vi "Ramp to Zero.vi"(6 "Axis":T1, 8 "error in (no error)":errorcluster, 11 "Instrument.VRM in":refnum<class "Instrument.OxfordVRM.lvclass">) -> (0 "error out":errorcluster, 2 "Response":string, 3 "Instrument.VRM out":refnum<class "Instrument.OxfordVRM.lvclass">)   [LabVIEW 2019, in "Instrument.OxfordVRM.lvclass"]
uses:
  Instrument.OxfordVRM.lvclass
  C:/Program Files (x86)/National Instruments/LabVIEW 2019/user.lib/LevyLab/Levylab Instruments/SMOs/Instrument/Instrument.lvclass
  Typedefs/VRM Magnet Axis--Enum.ctl
  <instrlib>/Mercury iXX/Public/Libraries/Magnet/Controls/PSU Actions.ctl
  Typedefs/Instrument.VRM.Commands-enum.ctl
  Typedefs/VRM Action-Axis--Cluster.ctl
  <userlib>/LevyLab/Instrument Framework/SMOs/Instrument/Instrument.lvclass/Instrument.ctl
  c467e4a8-4b58-44aa-8f24-0652f0f40db9.vi
  c467e4a8-4b58-44aa-8f24-0652f0f40db9.vi/cb162148-aced-4026-a92a-8c3683a6e699.vi
  c467e4a8-4b58-44aa-8f24-0652f0f40db9.vi/cb162148-aced-4026-a92a-8c3683a6e699.vi/90903bc8-b2cf-450b-a3a9-0f5a5b9220d8.vi
  <userlib>/LevyLab/Instrument Framework/SMOs/Instrument/API/Send and Receive.vi
  c467e4a8-4b58-44aa-8f24-0652f0f40db9.vi/cb162148-aced-4026-a92a-8c3683a6e699.vi/90903bc8-b2cf-450b-a3a9-0f5a5b9220d8.vi/98039df1-7789-4232-8489-3644d3569676.vi
  c467e4a8-4b58-44aa-8f24-0652f0f40db9.vi/cb162148-aced-4026-a92a-8c3683a6e699.vi/90903bc8-b2cf-450b-a3a9-0f5a5b9220d8.vi/acf00810-0388-4f91-a2e6-f9b1b5e55ebd.vi
  <userlib>/LevyLab/Instrument Framework/SMOs/Instrument/API/Enum to String.vi
  <userlib>/LevyLab/Instrument Framework/SMOs/RemoteControl/API/Send and Receive.vi
  <vilib>/Utility/Data Type/Get Type Information.vi
  <vilib>/JDP Science/JSONtext/JSON text to Variant.vi
  <vilib>/JDP Science/JSONtext/LVClass Serializer/JSONtext LVClass Serializer.lvclass
  <instrlib>/Mercury iXX/Public/Libraries/Magnet.lvlib
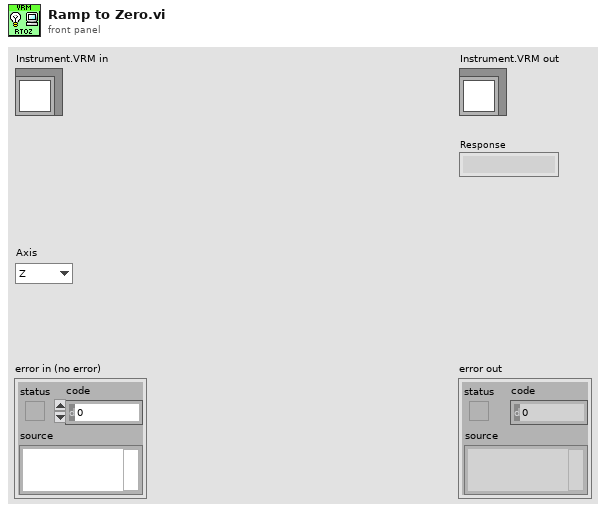
[diagram p1: front panel]
types:
  T1 = typedef "Instrument.OxfordVRM.lvclass/VRM Magnet Axis--Enum.ctl" = enum16{"Z", "X", "Y", "ALL"}
  T2 = typedef "Instrument.OxfordVRM.lvclass/VRM Action-Axis--Cluster.ctl" = cluster{"PSU Act Stat":T3, "Axis":T1}
  T3 = typedef "Mercury iXX.lvlib/Magnet.lvlib/PSU Actions.ctl" = string
  T4 = typedef "Instrument.OxfordVRM.lvclass/Instrument.VRM.Commands-enum.ctl" = enum16{"setAction", "setTarget", "setMagnetField", "getStatus", "getTarget", "getMagnetField"}
  T5 = cluster{"Holding":bool, "Ramp to Setpoint":bool, "Ramp to Zero":bool, "Clamp":bool}
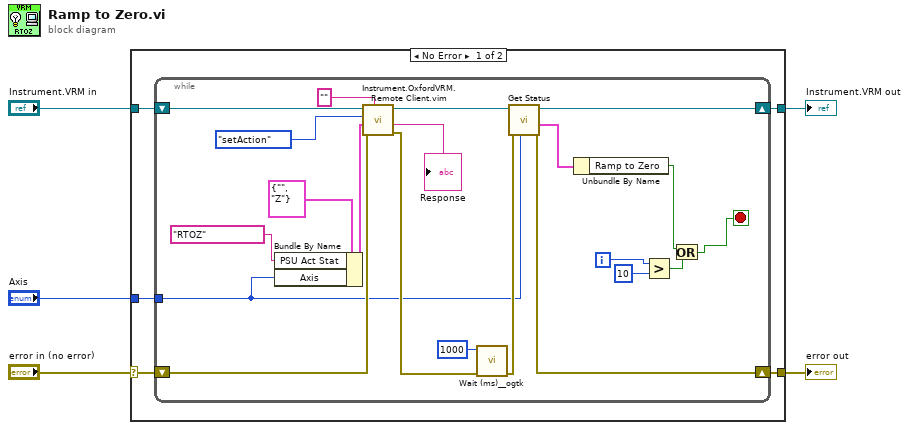
[diagram p0: block diagram]
diagram:
  n1 = case shown="No Error" "error in (no error)" {
    selector: "error in (no error)" -> [w9 w33]
    tunnel: [w7 w33] -> w4
    tunnel: [w8 w32] -> w2
    tunnel: "Instrument.VRM in" -> [w10 w32]
    tunnel: "Axis" -> [w6 _]
    frame No Error {
      n2 = while {
        shift-right: [w28] -> w8
        shift-left: w10 -> [w25]
        shift-right: [w26] -> w7
        shift-left: w9 -> [w31]
        tunnel: w6 -> [w13]
        i -> [w19]
        stop <- w21 stop-if-true
        n3 = Bundle By Name(cluster=T2 {"PSU Act Stat"="", "Axis"=enum."Z"}, "PSU Act Stat"=T3 "RTOZ", "Axis"=w13) -> (w15:T2)
        n4 = call "Instrument.OxfordVRM.Remote Client.vim"("Data Out type"="", "error in (no error)"=w31, "Data"=w15, "Commands"=Instrument.VRM.Commands-enum."setAction", "Instrument.VRM in"=w25) -> ("error out"=w18:errorcluster, "Data out"=→"Response":string, "Instrument.VRM out"=w20:refnum<class "Instrument.OxfordVRM.lvclass">)  [unwired: 4 in]
        n5 = call <userlib>:"Wait (ms)__ogtk.vi"("error in (no error)"=w18, "milliseconds to wait"=u32 1000) -> ("error out"=w27:errorcluster)  [unwired: 8 in, 1 out]
        n6 = call "Get Status.vi"("Axis"=w13, "error in (no error)"=w27, "Instrument.VRM in"=w20) -> ("error out"=w26:errorcluster, "Status (ALL)"=w29:T5, "Instrument.VRM out"=w28:refnum<class "Instrument.OxfordVRM.lvclass">)  [unwired: 5 in, 1 out]
        n7 = Unbundle By Name(w29) -> ("Ramp to Zero"=w22:bool)
        n8 = Greater?(x=w19, y=10) -> (0:w23:bool)
        n9 = Or(x=w22, y=w23) -> (x .or. y?=w21:bool)
      }
    }
    frame Error {
    }
  }
  "error out" <- w4
  "Instrument.VRM out" <- w2
